vi "AAL Resample (const to variable, complex multi-channel).vi"(7 "reset? (True)":bool=TRUE, 8 "error in (no error)":errorcluster, 9 "config":T1={"timing jitter"=enum."Interpolation", "anti-aliasing?"=TRUE, "filter prototype"={"coefficients"=[], "factor"=1}} {"filter prototype"."coefficients" format="%.2f"}, 10 "time":dbl[](array[numeric]) format="%.2f", 11 "X":cdb[][](array[numeric])) -> (0 "error out":errorcluster, 1 "offset":i64, 2 "time stamps":dbl[](array[numeric]) format="%.2f", 3 "Y":cdb[][](array[numeric]) format="%.2f")   [LabVIEW 2014, in "NI_AALPro.lvlib"]
doc: "Perform an arbitrary resampling on the input signal."
uses:
  NI_AALPro.lvlib
  lvanlys.dll
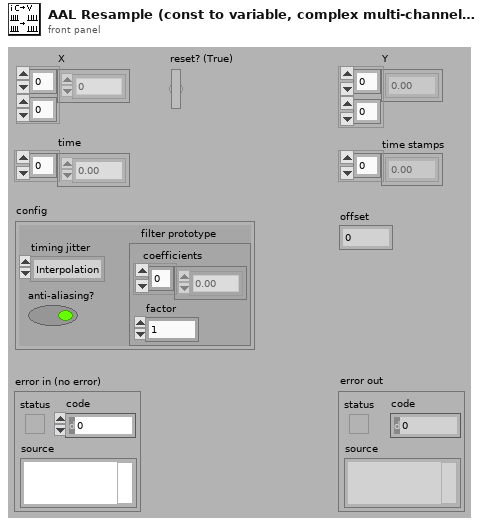
[diagram p1: front panel]
types:
  T1 = cluster{"timing jitter":enum32{"Interpolation", "Rounding"}, "anti-aliasing?":bool, "filter prototype":cluster{"coefficients":dbl[], "factor":i32}}
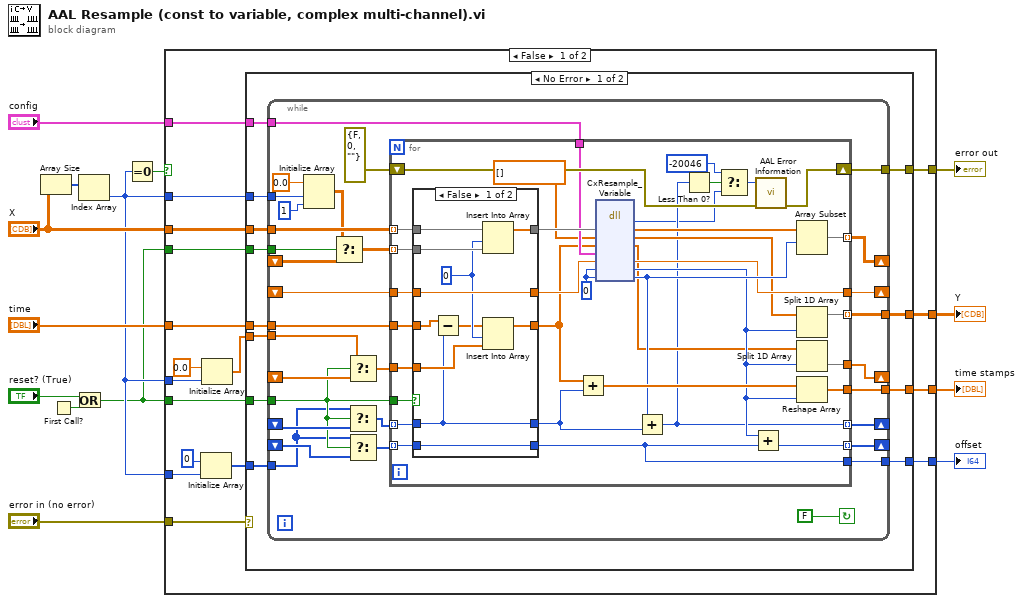
[diagram p0: block diagram]
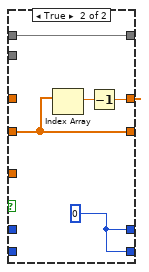
[diagram p2: hidden frame]
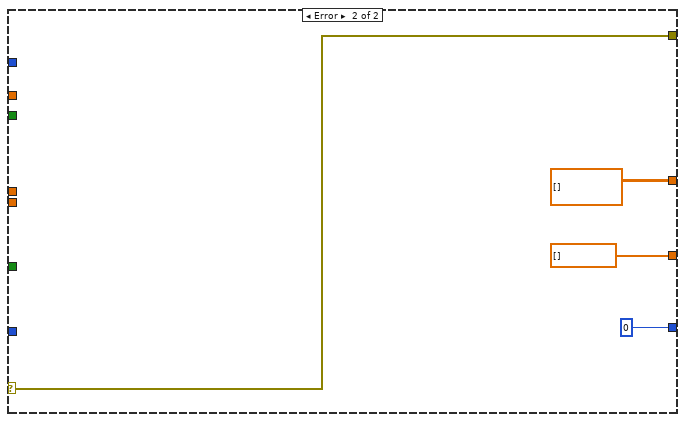
[diagram p3: hidden frame]
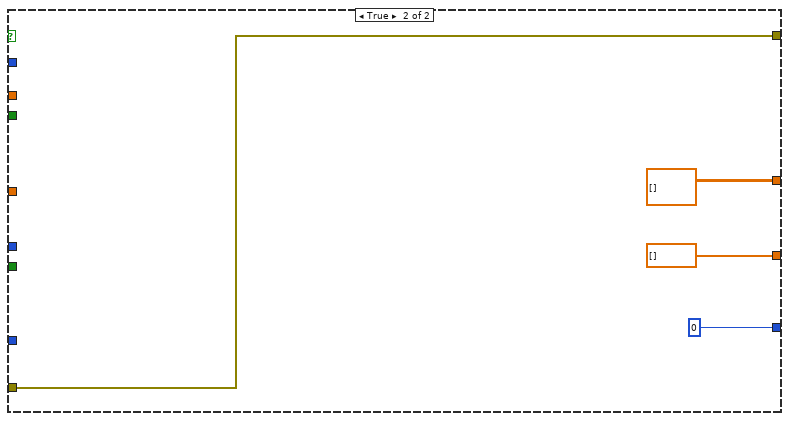
[diagram p4: hidden frame]
diagram:
  n1 = Array Size(array="X") -> (size(s)=w6:i32[])
  n2 = First Call?() -> (First Call?: T/F=w5:bool)
  n3 = Or(x="reset? (True)", y=w5) -> (x .or. y?=w1:bool)
  n4 = Index Array(array=w6) -> (element=w2:i32)  [unwired: 1 in]
  n5 = Equal To 0?(x=w2) -> (x = 0?=w3:bool)
  n6 = case shown="False" w3 {
    tunnel: "config" -> [w31 _]
    tunnel: "time" -> [w30 _]
    tunnel: [w29 dbl[] []] -> w12
    tunnel: [w28 dbl[][] []] -> w11
    tunnel: [w27 i64 0 ("element")] -> w10
    tunnel: [w26 w131] -> w9
    tunnel: "error in (no error)" -> [w25 w131]
    tunnel: "X" -> [w24 _]
    tunnel: w1 -> [w21 _]
    tunnel: w2 -> [w19 _]
    tunnel: w2 -> [w17 _]
    tunnel: w2 -> [w16 _]
    tunnel: w1 -> [w15 _]
    frame False {
      n7 = Initialize Array(i64 0 ("element"), w16) -> (w18:i64[])
      n8 = Initialize Array(0.0 ("element"), w17) -> (w20:dbl[])
      n9 = case shown="No Error" w25 {
        selector: w25 -> [_ w129]
        tunnel: w31 -> [w43 _]
        tunnel: w30 -> [w38 _]
        tunnel: [w42 dbl[] []] -> w29
        tunnel: [w41 cdb[][] []] -> w28
        tunnel: [w40 i64 0] -> w27
        tunnel: [w39 w129] -> w26
        tunnel: w24 -> [w37 _]
        tunnel: w21 -> [w36 _]
        tunnel: w19 -> [w35 _]
        tunnel: w15 -> [w34 _]
        tunnel: w20 -> [w33 _]
        tunnel: w18 -> [w32 _]
        frame No Error {
          n10 = while {
            tunnel: [w66] -> w41
            tunnel: [w62] -> w42
            shift-right: [w72] -> _
            shift-left: _ -> [w52]
            shift-right: [w73] -> _
            shift-left: _ -> [w57]
            tunnel: w37 -> [w69]
            tunnel: w38 -> [w68]
            shift-right: [w71] -> _
            shift-left: _ -> [w67]
            tunnel: w36 -> [w45]
            tunnel: w43 -> [w74]
            shift-right: [w65] -> _
            shift-left: _ -> [w46]
            tunnel: [w64] -> w40
            shift-right: [w63] -> _
            shift-left: _ -> [w48]
            tunnel: [w60] -> w39
            tunnel: w34 -> [w58]
            tunnel: w35 -> [w53]
            tunnel: w33 -> [w50]
            tunnel: w32 -> [w44]
            stop <- FALSE continue-if-true
            n11 = Initialize Array(0.0, w53, 1 ("dimension size")) -> (w54:dbl[][])
            n12 = Select(t=w54, s=w58, f=w57) -> (s? t:f=w59:cdb[][])
            n13 = Select(t=w50, s=w45, f=w52) -> (s? t:f=w51:dbl[])
            n14 = Select(t=w44, s=w45, f=w46) -> (s? t:f=w47:i64[])
            n15 = Select(t=w44, s=w45, f=w48) -> (s? t:f=w49:i64[])
            n16 = for {
              tunnel: w74 -> [w86]
              tunnel: [w109] -> w73 mode=indexing
              tunnel: [w80] -> w72
              tunnel: [w88] -> w71
              tunnel: w69 -> [w108] mode=indexing
              tunnel: w68 -> [w106]
              tunnel: w59 -> [w105] mode=indexing
              tunnel: w51 -> [w104]
              tunnel: w67 -> [w103]
              tunnel: w45 -> [w102]
              tunnel: w47 -> [w101] mode=indexing
              tunnel: [w100] -> w66 mode=indexing
              tunnel: [w76] -> w65 mode=indexing
              tunnel: w49 -> [w97] mode=indexing
              tunnel: [w95] -> w64
              tunnel: [w94] -> w63 mode=indexing
              tunnel: [w93] -> w62
              shift-right: [w91] -> w60
              shift-left: errorcluster {"status"=FALSE, "code"=0, "source"=""} ("error out") -> [w92]
              w90 = 0
              n17 = case shown="False" w102 {
                tunnel: [w119 w125] -> w107
                tunnel: w108 -> [w117 w125]
                tunnel: [w114 w124] -> w84
                tunnel: w106 -> [w113 w124]
                tunnel: [w120 w122] -> w87
                tunnel: w105 -> [w116 _]
                tunnel: w104 -> [w118 _]
                tunnel: w103 -> [w120 _]
                tunnel: w101 -> [w111 _]
                tunnel: [w111 w121] -> w96
                tunnel: w97 -> [w110 _]
                tunnel: [w110 w121] -> w95
                frame False {
                  w115 = 0 ("Index")
                  n18 = Subtract(x=w113, y=w111) -> (x-y=w112:dbl[])
                  n19 = Insert Into Array(array=w117, index=w115, new element=w116) -> (w119:cdb[])
                  n20 = Insert Into Array(array=w112, index=w115, new element=w118) -> (w114:dbl[])
                }
                frame True {
                  w121 = i64 0
                  n21 = Index Array(array=w124) -> (element=w123:dbl)  [unwired: 1 in]
                  n22 = Decrement(x=w123) -> (x-1=w122:dbl)
                }
              }
              n23 = Add(x=w84, y=w96) -> (x+y=w99:dbl[])
              n24 = dll-call lib="C:/Program Files (x86)/National Instruments/LabVIEW 2014/resource/lvanlys.*" fn="CxResample_Variable"("X"=w107, "X"=cdb[] [], "timeH"=w84, "config"=w86, "last_sample_time"=w87, "out_len"=w90, "xLeftOverIdx"=w90) -> (w75:i32, "X"=w98:cdb[], "X"=w85:cdb[], "timeH"=w81:dbl[], "last_sample_time"=w88:dbl, "out_len"=w82:i32, "xLeftOverIdx"=w89:i32)  [unwired: 4 in, 2 out]
              n25 = Add(x=w89, y=w96) -> (x+y=w76:i64)
              n26 = Less Than 0?(x=w76) -> (x < 0?=w79:bool)
              n27 = Select(t=-20046 ("error"), s=w79, f=w75) -> (s? t:f=w77:i32)
              n28 = Add(x=w82, y=w95) -> (x+y=w94:i64)
              n29 = call "AAL Error Information.vi"("error in (no error)"=w92, "error code"=w77) -> ("error out"=w91:errorcluster)  [unwired: 9 in]
              n30 = Array Subset(array=w98, index=w89) -> (w109:cdb[])  [unwired: 1 in]
              n31 = Split 1D Array(array=w85, index=w82) -> (first subarray=w100:cdb[])  [unwired: 1 out]
              n32 = Split 1D Array(array=w81, index=w82) -> (second subarray=w80:dbl[])  [unwired: 1 out]
              n33 = Reshape Array(w99, w82) -> (w93:dbl[])
            }
          }
        }
        frame Error {
        }
      }
    }
    frame True {
    }
  }
  "time stamps" <- w12
  "Y" <- w11
  "offset" <- w10
  "error out" <- w9
